vi "io_attr_query.vi"(5 "Query Parameter (None)":string, 7 "Attribute":T1={"Identifier"="", "Descriptive Name"="", "Data Type"=enum."Integer 32", "Command"="", "Access"=enum."Read/Write", "Range Table"="", "Read Callback"="", "Write Callback"="", "Supported Models"="", "Instrument Options"="", "Index"=0, "OPC Wait"=FALSE, "No Status Check"=FALSE, "Cache Only"=FALSE}, 8 "error in":errorcluster caption="error in (no error)", 10 "write buffer":string, 11 "VISA resource name":refnum<visa-resource-name>) -> (0 "error out":errorcluster, 2 "read buffer":string, 3 "VISA resource name out":refnum<visa-resource-name>)   [LabVIEW 2022 SP3, in "hmp4000_rsidr_core.lvlib"]
uses:
  hmp4000_rsidr_core.lvlib
  type_Attribute.ctl
  type_Attribute_Data_Type.ctl
  type_ReadWriteAccess.ctl
  _type_Operation_Fgv_RangeTable.ctl
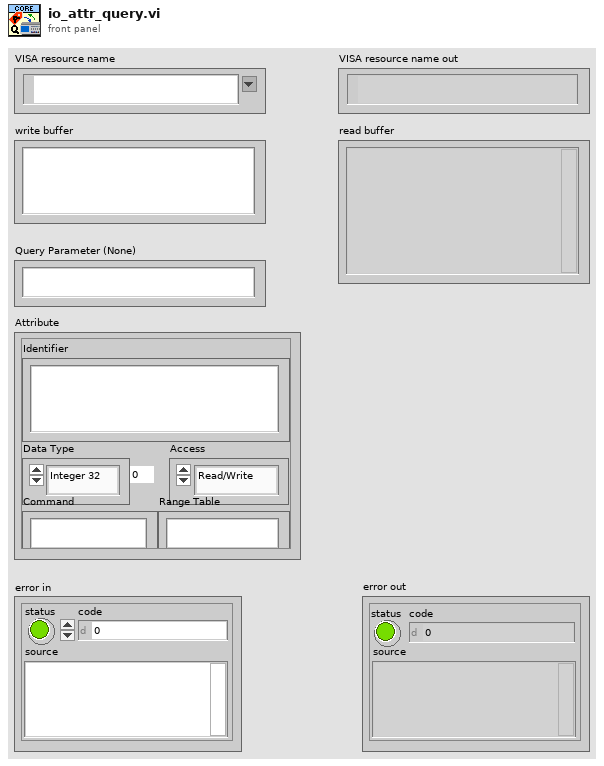
[diagram p1: front panel]
types:
  T1 = typedef "hmp4000_rsidr_core.lvlib/type_Attribute.ctl" = cluster{"Identifier":string, "Descriptive Name":string, "Data Type":T2, "Command":string, "Access":T3, "Range Table":string, "Read Callback":string, "Write Callback":string, "Supported Models":string, "Instrument Options":string, "Index":i32, "OPC Wait":bool, "No Status Check":bool, "Cache Only":bool}
  T2 = typedef "hmp4000_rsidr_core.lvlib/type_Attribute_Data_Type.ctl" = enum16{"Integer 32", "Double", "String", "Boolean", "None", "Integer 64", "RawString"}
  T3 = typedef "hmp4000_rsidr_core.lvlib/type_ReadWriteAccess.ctl" = enum16{"Read Only", "Write Only", "Read/Write"}
  T4 = typedef "hmp4000_rsidr_core.lvlib/_type_Operation_Fgv_RangeTable.ctl" = enum16{"Initialize", "Check", "Coerce", "Get Command String", "Get Numeric Value", "Get Default Value", "Get Range Table Type"}
  T5 = typedef "hmp4000_rsidr_core.lvlib/type_Session_Data.ctl" = cluster{"IDN string":string, "Instrument FW":string, "Instr type":string, "Instr type for err. msg.":string, "Installed Options":string[], "Ignore Error Messages":string, "Logging params":variant, "OPC Timeout":i32, "VISA Timeout":i32, "STB Poll VISA Timeout":i32, "Additional Flags":i32, "Wait Before Read":i32, "Wait Before Write":i32, "Option String Flags":i32, "IO Segment Size":i64, "VISA Access Mode":T6, "Interface Type":T7, "OPC Wait Mode":T8, "Bin Float Number  Format":T9, "Bin Integer Number Format":T10, "Simulate":bool, "VXIcapable":bool, "Duplicate Session":bool, "Add LF to Write":bool, "Logging":bool, "Fast Sweep":bool, "Query Instrument Status":bool, "Check Range":bool, "Check Options":bool}
  T6 = typedef "hmp4000_rsidr_core.lvlib/type_VisaAccessMode.ctl" = u16
  T7 = typedef "hmp4000_rsidr_core.lvlib/type_InterfaceType.ctl" = enum16{"Unknown", "GPIB", "VXI", "GPIB_VXI", "ASRL", "PXI", "TCPIP", "USB", "SOCKET"}
  T8 = typedef "hmp4000_rsidr_core.lvlib/type_OPC_Wait_Mode.ctl" = enum16{"STBpolling", "STBpollingSlow", "STBpollingSuperSlow", "ServiceRequest", "OPCquery"}
  T9 = typedef "hmp4000_rsidr_core.lvlib/type_Binary_Float_Number_Format.ctl" = enum16{"Float_4_Bytes_Swapped", "Float_4_Bytes", "Double_8_Bytes_Swapped", "Double_8_Bytes"}
  T10 = typedef "hmp4000_rsidr_core.lvlib/type_Binary_Integer_Number_Format.ctl" = enum16{"Int32_4_Bytes_Swapped", "Int32_4 Bytes", "Int16_2_Bytes_Swapped", "Int16_2_Bytes"}
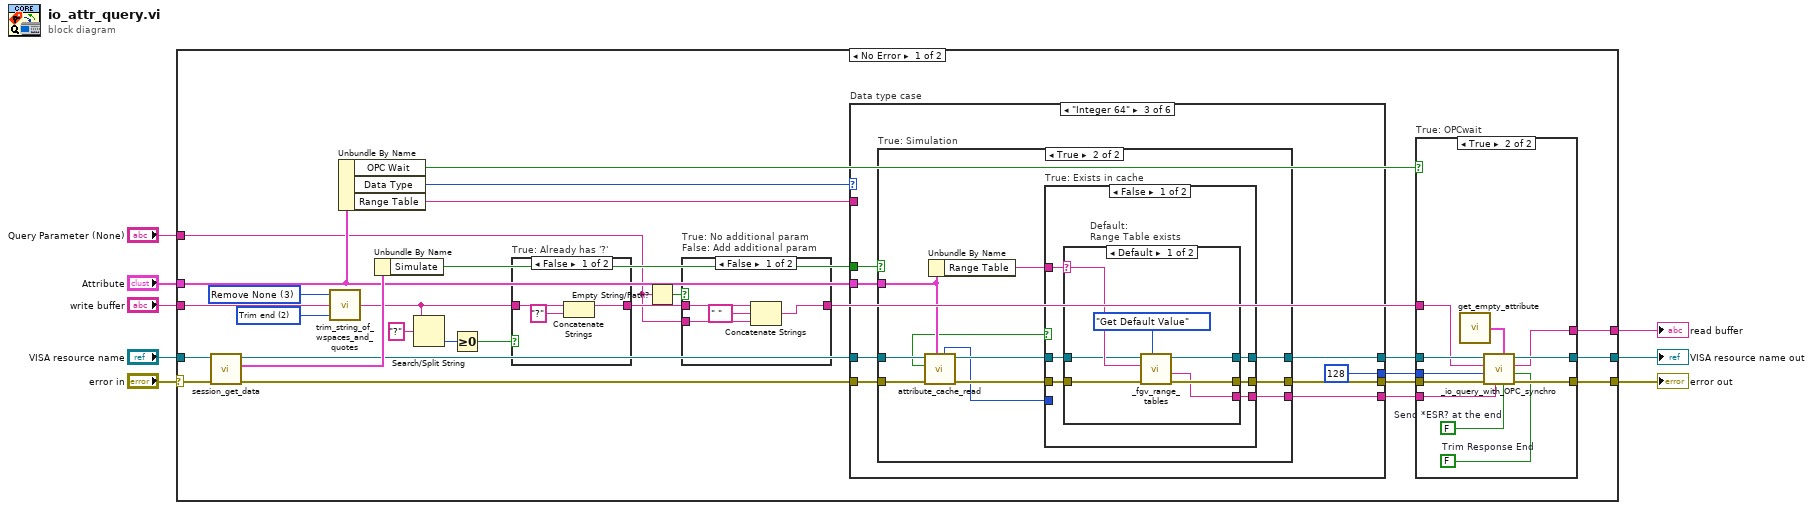
[diagram p0: block diagram]
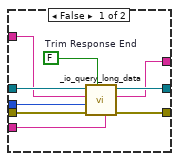
[diagram p3: hidden frame]
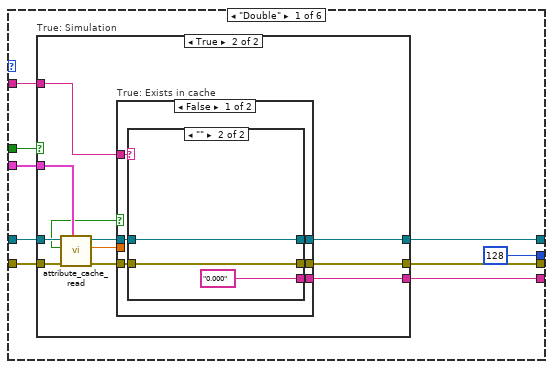
[diagram p5: hidden frame]
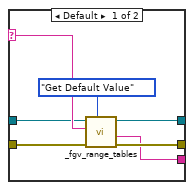
[diagram p7: hidden frame]
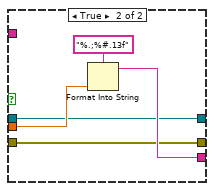
[diagram p8: hidden frame]
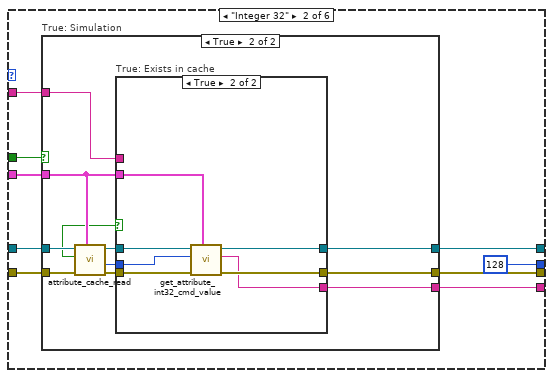
[diagram p9: hidden frame]
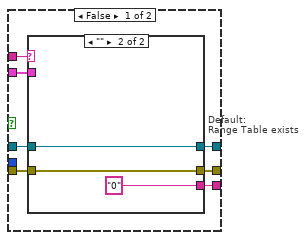
[diagram p11: hidden frame]
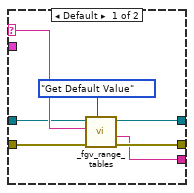
[diagram p12: hidden frame]
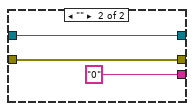
[diagram p14: hidden frame]
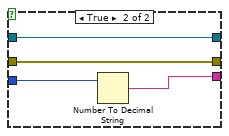
[diagram p15: hidden frame]
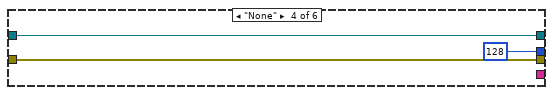
[diagram p16: hidden frame]
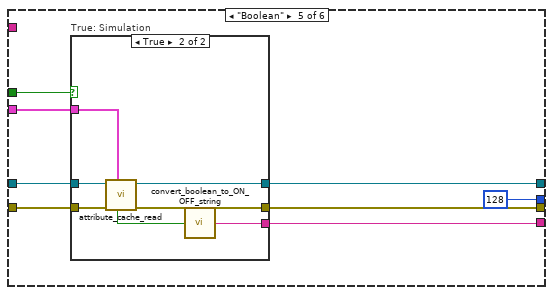
[diagram p17: hidden frame]
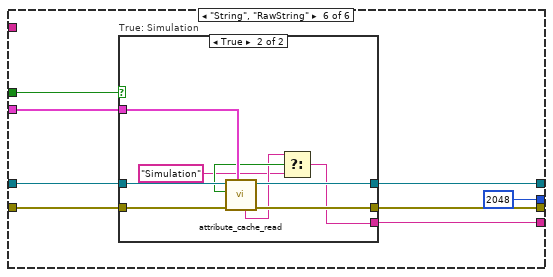
[diagram p19: hidden frame]
diagram:
  n1 = case shown="No Error" "error in" {
    selector: "error in" -> [w33 w236]
    tunnel: "VISA resource name" -> [w32 w235]
    tunnel: [w17 w236] -> w3
    tunnel: [w16 w235] -> w2
    tunnel: [w13 _] -> w8
    tunnel: "write buffer" -> [w26 _]
    tunnel: "Attribute" -> [w31 _]
    tunnel: "Query Parameter (None)" -> [w10 _]
    frame No Error {
      w23 = u16 3 items=["Remove All Quotes", "Remove Single Quotes", "Remove Double Quotes", "Remove None"] ("Remove quotes (Remove All)")
      w25 = u16 2 items=["Trim both", "Trim start", "Trim end", "Trim none"] ("Trim whitespaces (Trim both)")
      n2 = call "session_get_data.vi"("error in"=w33, "VISA resource name"=w32) -> ("error out"=w21:errorcluster, "Session User Data out"=w36:T5, "VISA resource name out"=w22:refnum<visa-resource-name>)  [unwired: 6 in, 1 out]
      n3 = call "trim_string_of_wspaces_and_quotes.vi"("Trim whitespaces (Trim both)"=w25, "String in"=w26, "Remove quotes (Remove All)"=w23) -> ("String out"=w24:string)  [unwired: 2 in]
      n4 = Unbundle By Name(w31) -> ("OPC Wait"=w20:bool, "Data Type"=w35:T2, "Range Table"=w27:string)
      n5 = Unbundle By Name(w36) -> ("Simulate"=w34:bool)
      n6 = Search/Split String(string=w24, search string/char (-)="?" ("string")) -> (offset of match=w29:i32)  [unwired: 1 in, 2 out]
      n7 = Greater Or Equal To 0?(x=w29) -> (x >= 0?=w28:bool)
      n8 = case "True: Already has '?'" shown="False" w28 {
        tunnel: w24 -> [w64 w65]
        tunnel: [w62 w65] -> w11
        frame False {
          n9 = Concatenate Strings(w64, "?" ("string")) -> (w62:string)
        }
        frame True {
        }
      }
      n10 = Empty String/Path?(string/path=w10) -> (empty?=w12:bool)
      n11 = case "True: No additional param\nFalse: Add additional param" shown="False" w12 {
        tunnel: w11 -> [w38 w41]
        tunnel: [w37 w41] -> w9
        tunnel: w10 -> [w39 _]
        frame False {
          n12 = Concatenate Strings(w38, " " ("string"), w39) -> (w37:string)
        }
        frame True {
        }
      }
      n13 = case "Data type case" shown="\"Integer 64\"" w35 {
        tunnel: w21 -> [w73 w116 w160 w197 w205 w222]
        tunnel: w22 -> [w72 w115 w159 w198 w204 w221]
        tunnel: [w67 w111 w157 w197 w201 w218] -> w19
        tunnel: [w68 w112 w158 w198 w202 w219] -> w18
        tunnel: w34 -> [w74 w117 w161 _ w206 w223]
        tunnel: w31 -> [w71 w113 w162 _ w203 w220]
        tunnel: w27 -> [w70 w114 _ _ _ _]
        tunnel: [w69 w110 w156 _ w200 w217] -> w15
        tunnel: [u32 128 u32 128 u32 128 u32 128 u32 128 u32 2048] -> w14
        frame "Double" {
          n14 = case "True: Simulation" shown="True" w74 {
            tunnel: w73 -> [w76 w87]
            tunnel: w72 -> [w75 w86]
            tunnel: [w75 w79] -> w68
            tunnel: [w76 w83] -> w67
            tunnel: w71 -> [_ w82]
            tunnel: [_ w77] -> w69
            tunnel: w70 -> [_ w78]
            frame False {
            }
            frame True {
              n15 = call "attribute_cache_read.vi"("Attribute"=w82, "error in"=w87, "VISA resource name"=w86) -> ("error out"=w85:errorcluster, "Double out"=w84:dbl, "VISA resource name out"=w80:refnum<visa-resource-name>, "Exists in cache"=w81:bool)  [unwired: 1 in, 4 out]
              n16 = case "True: Exists in cache" shown="False" w81 {
                tunnel: w85 -> [w91 w105]
                tunnel: w84 -> [_ w106]
                tunnel: [w90 w105] -> w83
                tunnel: [w92 w107] -> w77
                tunnel: w78 -> [w93 _]
                tunnel: w80 -> [w89 w104]
                tunnel: [w88 w104] -> w79
                frame False {
                  n17 = case shown="\"\"" w93 {
                    selector: w93 -> [w98 _]
                    tunnel: [w94 "0.000"] -> w92
                    tunnel: w91 -> [w100 w102]
                    tunnel: [w99 w102] -> w90
                    tunnel: w89 -> [w97 w101]
                    tunnel: [w96 w101] -> w88
                    frame Default {
                      n18 = call "_fgv_range_tables.vi"("Operation"=_type_Operation_Fgv_RangeTable."Get Default Value", "error in"=w100, "Range Table ID in"=w98, "VISA resource name"=w97) -> ("error out"=w99:errorcluster, "String Value out"=w94:string, "VISA resource name out"=w96:refnum<visa-resource-name>)  [unwired: 3 in, 2 out]
                    }
                    frame "" {
                    }
                  }
                }
                frame True {
                  n19 = Format Into String(format string="%.;%#.13f", w106) -> (resulting string=w107:string)  [unwired: 2 in, 1 out]
                }
              }
            }
          }
        }
        frame "Integer 32" {
          n20 = case "True: Simulation" shown="True" w117 {
            tunnel: w116 -> [w119 w130]
            tunnel: w115 -> [w118 w129]
            tunnel: [w118 w122] -> w112
            tunnel: [w119 w127] -> w111
            tunnel: w113 -> [_ w128]
            tunnel: [_ w120] -> w110
            tunnel: w114 -> [_ w121]
            frame False {
            }
            frame True {
              n21 = call "attribute_cache_read.vi"("Attribute"=w128, "error in"=w130, "VISA resource name"=w129) -> ("error out"=w125:errorcluster, "Int32 out"=w126:i32, "VISA resource name out"=w123:refnum<visa-resource-name>, "Exists in cache"=w124:bool)  [unwired: 1 in, 4 out]
              n22 = case "True: Exists in cache" shown="True" w124 {
                tunnel: w121 -> [w137 _]
                tunnel: w128 -> [w136 w149]
                tunnel: [w135 w152] -> w127
                tunnel: w126 -> [_ w150]
                tunnel: w125 -> [w134 w154]
                tunnel: w123 -> [w133 w153]
                tunnel: [w132 w151] -> w122
                tunnel: [w131 w148] -> w120
                frame False {
                  n23 = case "Default:\nRange Table exists" shown="\"\"" w137 {
                    selector: w137 -> [w142 _]
                    tunnel: [w143 w147] -> w135
                    tunnel: w136 -> [_ _]
                    tunnel: w134 -> [w144 w147]
                    tunnel: w133 -> [w141 w146]
                    tunnel: [w140 w146] -> w132
                    tunnel: [w138 "0" ("String Value out")] -> w131
                    frame Default {
                      n24 = call "_fgv_range_tables.vi"("Operation"=_type_Operation_Fgv_RangeTable."Get Default Value", "error in"=w144, "Range Table ID in"=w142, "VISA resource name"=w141) -> ("error out"=w143:errorcluster, "String Value out"=w138:string, "VISA resource name out"=w140:refnum<visa-resource-name>)  [unwired: 3 in, 2 out]
                    }
                    frame "" {
                    }
                  }
                }
                frame True {
                  n25 = call "get_attribute_int32_cmd_value.vi"("Attribute"=w149, "error in"=w154, "Input Int32 value"=w150, "VISA resource name"=w153) -> ("error out"=w152:errorcluster, "Cmd Value out"=w148:string, "VISA resource name out"=w151:refnum<visa-resource-name>)  [unwired: 5 in]
                }
              }
            }
          }
        }
        frame "Integer 64" {
          n26 = case "True: Simulation" shown="True" w161 {
            tunnel: w160 -> [w164 w175]
            tunnel: w159 -> [w163 w174]
            tunnel: [w163 w167] -> w158
            tunnel: [w164 w171] -> w157
            tunnel: w162 -> [_ w172]
            tunnel: [_ w166] -> w156
            frame False {
            }
            frame True {
              n27 = call "attribute_cache_read.vi"("Attribute"=w172, "error in"=w175, "VISA resource name"=w174) -> ("error out"=w170:errorcluster, "VISA resource name out"=w168:refnum<visa-resource-name>, "Int64 out"=w165:i64, "Exists in cache"=w169:bool)  [unwired: 1 in, 4 out]
              n28 = Unbundle By Name(w172) -> ("Range Table"=w173:string)
              n29 = case "True: Exists in cache" shown="False" w169 {
                tunnel: w173 -> [w181 _]
                tunnel: [w180 w194] -> w171
                tunnel: [w179 w195] -> w166
                tunnel: w165 -> [_ w192]
                tunnel: w170 -> [w178 w194]
                tunnel: w168 -> [w177 w193]
                tunnel: [w176 w193] -> w167
                frame False {
                  n30 = case "Default:\nRange Table exists" shown="Default" w181 {
                    selector: w181 -> [w186 _]
                    tunnel: [w187 w191] -> w180
                    tunnel: [w182 "0"] -> w179
                    tunnel: w178 -> [w188 w191]
                    tunnel: w177 -> [w185 w189]
                    tunnel: [w184 w189] -> w176
                    frame Default {
                      n31 = call "_fgv_range_tables.vi"("Operation"=_type_Operation_Fgv_RangeTable."Get Default Value", "error in"=w188, "Range Table ID in"=w186, "VISA resource name"=w185) -> ("error out"=w187:errorcluster, "String Value out"=w182:string, "VISA resource name out"=w184:refnum<visa-resource-name>)  [unwired: 3 in, 2 out]
                    }
                    frame "" {
                    }
                  }
                }
                frame True {
                  n32 = Number To Decimal String(number=w192) -> (decimal integer string=w195:string)  [unwired: 1 in]
                }
              }
            }
          }
        }
        frame "None" {
        }
        frame "Boolean" {
          n33 = case "True: Simulation" shown="True" w206 {
            tunnel: w205 -> [w208 w215]
            tunnel: w204 -> [w207 w214]
            tunnel: [w207 w213] -> w202
            tunnel: [w208 w211] -> w201
            tunnel: w203 -> [_ w212]
            tunnel: [_ w209] -> w200
            frame False {
            }
            frame True {
              n34 = call "attribute_cache_read.vi"("Attribute"=w212, "error in"=w215, "VISA resource name"=w214) -> ("error out"=w211:errorcluster, "VISA resource name out"=w213:refnum<visa-resource-name>, "Boolean out"=w210:bool)  [unwired: 1 in, 5 out]
              n35 = call "convert_boolean_to_ON_OFF_string.vi"("boolean value in"=w210) -> ("string value out"=w209:string)  [unwired: 4 in]
            }
          }
        }
        frame "String", "RawString" {
          n36 = case "True: Simulation" shown="True" w223 {
            tunnel: w222 -> [w225 w234]
            tunnel: w221 -> [w224 w233]
            tunnel: [w224 w232] -> w219
            tunnel: [w225 w230] -> w218
            tunnel: w220 -> [_ w231]
            tunnel: [_ w229] -> w217
            frame False {
            }
            frame True {
              n37 = call "attribute_cache_read.vi"("Attribute"=w231, "error in"=w234, "VISA resource name"=w233) -> ("error out"=w230:errorcluster, "VISA resource name out"=w232:refnum<visa-resource-name>, "String out"=w227:string, "Exists in cache"=w228:bool)  [unwired: 1 in, 4 out]
              n38 = Select(t=w227, s=w228, f="Simulation") -> (s? t:f=w229:string)
            }
          }
        }
      }
      n39 = case "True: OPCwait" shown="True" w20 {
        tunnel: w19 -> [w50 w61]
        tunnel: w18 -> [w49 w60]
        tunnel: [w48 w59] -> w17
        tunnel: [w47 w58] -> w16
        tunnel: w9 -> [w45 w53]
        tunnel: w15 -> [w43 w54]
        tunnel: w14 -> [w46 w57]
        tunnel: [w44 w56] -> w13
        frame False {
          w42 = FALSE  # Trim Response End
          n40 = call "_io_query_long_data.vi"("Simulation read buffer (\"Simulation\")"=w43, "Trim Response End"=w42, "error in"=w50, "Max chunk read bytes count (65536)"=w46, "Write buffer"=w45, "VISA resource name"=w49) -> ("error out"=w48:errorcluster, "Read buffer"=w44:string, "VISA resource name out"=w47:refnum<visa-resource-name>)  [unwired: 3 in]
        }
        frame True {
          w52 = FALSE  # Trim Response End
          w55 = FALSE  # Send *ESR? at the end
          n41 = call "get_empty_attribute.vi"() -> ("Empty Attribute out"=w51:T1)
          n42 = call "_io_query_with_OPC_synchro.vi"("Trim Response End"=w52, "Send *ESR? at the end (T)"=w55, "Attribute"=w51, "Simulation read buffer (\"Simulation\")"=w54, "error in"=w61, "Max segment read bytes count (65536)"=w57, "Query"=w53, "VISA resource name"=w60) -> ("error out"=w59:errorcluster, "Response"=w56:string, "VISA resource name out"=w58:refnum<visa-resource-name>)  [unwired: 1 in]
        }
      }
    }
    frame Error {
    }
  }
  "VISA resource name out" <- w2
  "error out" <- w3
  "read buffer" <- w8
